vi "Read All.vi"(8 "Error In":errorcluster) -> (0 "Error Out":errorcluster)   [LabVIEW 2018, in "Tests.lvlib" / "Readers.lvlib" / "String.lvlib"]
uses:
  String.lvlib
  src/Toolkit/Readers/String/String.lvclass
  <vilib>/addons/_JKI Toolkits/Caraya/classes/Test/Test.lvclass
  <vilib>/addons/_JKI Toolkits/Caraya/classes/Assert/Assert.lvclass
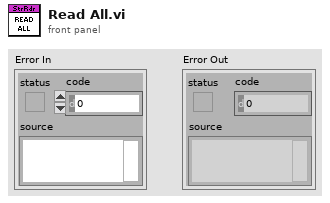
[diagram p1: front panel]
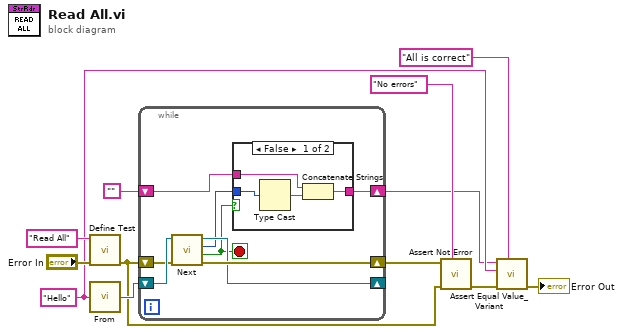
[diagram p0: block diagram]
diagram:
  w4 = "Hello" ("String")
  n1 = call <vilib>:"Define Test.vi"("error in (no error)"="Error In", "Label (VI Title)"="Read All") -> ("error out"=w1:errorcluster)  [unwired: 9 in]
  n2 = call "From.vi"("String"=w4) -> ("String"=w10:refnum<class "String.lvclass">)
  n3 = while {
    shift-right: [w18] -> w9
    shift-left: w1 -> [w19]
    shift-right: [w17] -> _
    shift-left: w10 -> [w20]
    shift-right: [w14] -> w2
    shift-left: "" -> [w15]
    stop <- w16 stop-if-true
    n4 = call-dynamic "Next.vi"("Error In"=w19, "Reader In"=w20) -> ("Error Out"=w18:errorcluster, "Done"=w16:bool, "Character"=w13:u8, "Reader Out"=w17:refnum<class "String.lvclass">)  [unwired: 6 in]
    n5 = case shown="False" w16 {
      tunnel: w15 -> [w24 w25]
      tunnel: [w23 w25] -> w14
      tunnel: w13 -> [w22 _]
      frame False {
        n6 = Type Cast(x=w22) -> (*(type *) &x=w21:string)  [unwired: 1 in]
        n7 = Concatenate Strings(w24, w21) -> (w23:string)
      }
      frame True {
      }
    }
  }
  n8 = call <vilib>:"Assert Not Error.vi"("Label"="No errors", "error in (no error)"=w1, "Not Error?"=w9) -> ("error out"=w7:errorcluster)  [unwired: 8 in]
  n9 = call <vilib>:"Assert Equal Value_Variant.vi"("Label"="All is correct", "error in (no error)"=w7, "Y"=w4, "X"=w2) -> ("error out"=→"Error Out":errorcluster)  [unwired: 7 in]
